vi "功率计测试平台.vi"(11 "Queue Ref In":T1={"UI"=refnum, "Message"=refnum, "Data"=refnum, "Caller"=refnum, "Name"="000 Common", "Data Path"=path "", "Class Path"=path "", "SubPanel"=refnum, "Project Name"="", "MNT"="", "Title"="", "Data Source"=refnum, "Queue List"={}, "VI"=refnum, "UE"=refnum}) -> ()   [LabVIEW 2020]
doc: "000001"
uses:
  Alin/QMH/000 Module Data Type.ctl
  Alin/QMH/Queue Message.ctl
  <vilib>/Utility/NIReport.llb/NI_report.lvclass
  <vilib>/Utility/NIReport.llb/Report Type.ctl
  <vilib>/addons/_office/excel.llb/Excel Easy Table (str).vi
  <vilib>/Utility/NIReport.llb/NI_ReportGenerationCore.lvlib
  <vilib>/Utility/NIReport.llb/Excel/NI_Excel.lvclass
  <vilib>/addons/_office/NI_ReportGenerationToolkit.lvlib
panel:
  out "SN:":string
  out "型号:":string
  in  "Connect":bool
  out "Connected?":bool
  in  "Port":u16 caption="Port:"
  in  "IP:":string
  out "消息":string
  in  "结束":bool
  in  "开始":bool
  in  "时间间隔(s)":dbl=1.0
  out "-W/mW":dbl format="%#.6f W"
  in  "反向通道Offset":dbl min=-60.0 max=60.0 format="%#.2f"
  out "驻波比":dbl format="%#.2f"
  in  "驻波比限值":dbl
  out "W/mW":dbl format="%#.6f W"
  in  "Write":bool
  in  "Read":bool
  in  "正向通道Offset":dbl min=-60.0 max=60.0 format="%#.2f"
  in  "Frequency":dbl=1.0 min=1.0 max=2.0 step=0.1 format="%#.1f GHz"
  out "Channel 1":dbl(knob) scale=0.0..60.0 scale format="%#_2f"
  out "Channel 2":dbl(knob) scale=0.0..60.0 scale format="%#_2f"
  # "Power-CHB"
  # "Power-CHA"
  # "dBm"
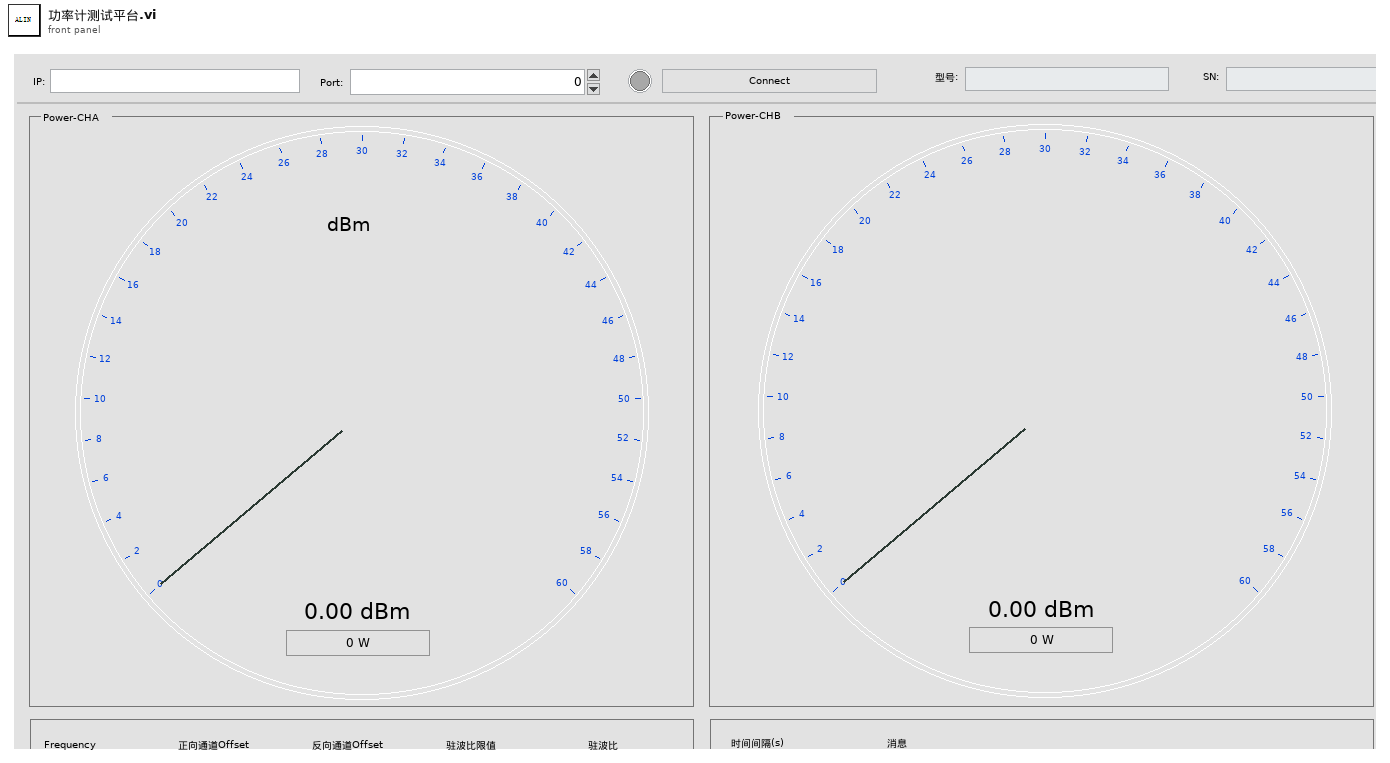
[diagram p1: front panel]
types:
  T1 = typedef "000 Module Data Type.ctl" = cluster{"UI":refnum<queue>, "Message":refnum<queue>, "Data":refnum<queue>, "Caller":refnum<queue>, "Name":string, "Data Path":path, "Class Path":path, "SubPanel":refnum<vi>, "Project Name":string, "MNT":string, "Title":string, "Data Source":refnum<queue>, "Queue List":map{string, refnum<queue>}, "VI":refnum<vi>, "UE":refnum<user-event>}
  T2 = cluster{"Queue":T1, "Delay":cluster{"Count Time(ms)":u32, "Delay Time(ms)":u32, "Next":string}, "connection ID":refnum<k5>, "Save path":path, "report":refnum<class "NI_report.lvclass">, "Count":u32}
  T3 = typedef "NI_ReportGenerationCore.lvlib/Report Type.ctl" = enum16{"HTML", "Word", "Excel"}
  T4 = enum16{"maximized", "minimized", "normal", "no change"}
  T5 = typedef "eventvkey.ctl" = enum16{"ASCII", "Enter", "Return", "Shift", "Ctrl", "Alt", "Cmd", "Opt", "Caps", "NumLock", "Clear", "Break", "Up", "Down", "Left", "Right", "Insert", "Delete", "Home", "End", "PageUp", "PageDown", "Escape", "Help", "Pause", "ScrollLock", "F1", "F2", "F3", "F4", "F5", "F6", "F7", "F8", "F9", "F10", "F11", "F12", "F13", "F14", "F15", "F16", "F17", "F18", "F19", "F20", "F21", "F22", "F23", "F24", "Play", "VolumeUp", "VolumeDown", "Mute", "Two Byte Char"}
  T6 = cluster{"Shift":bool, "Ctrl":bool, "Alt":bool, "Cmd":bool, "Opt":bool}
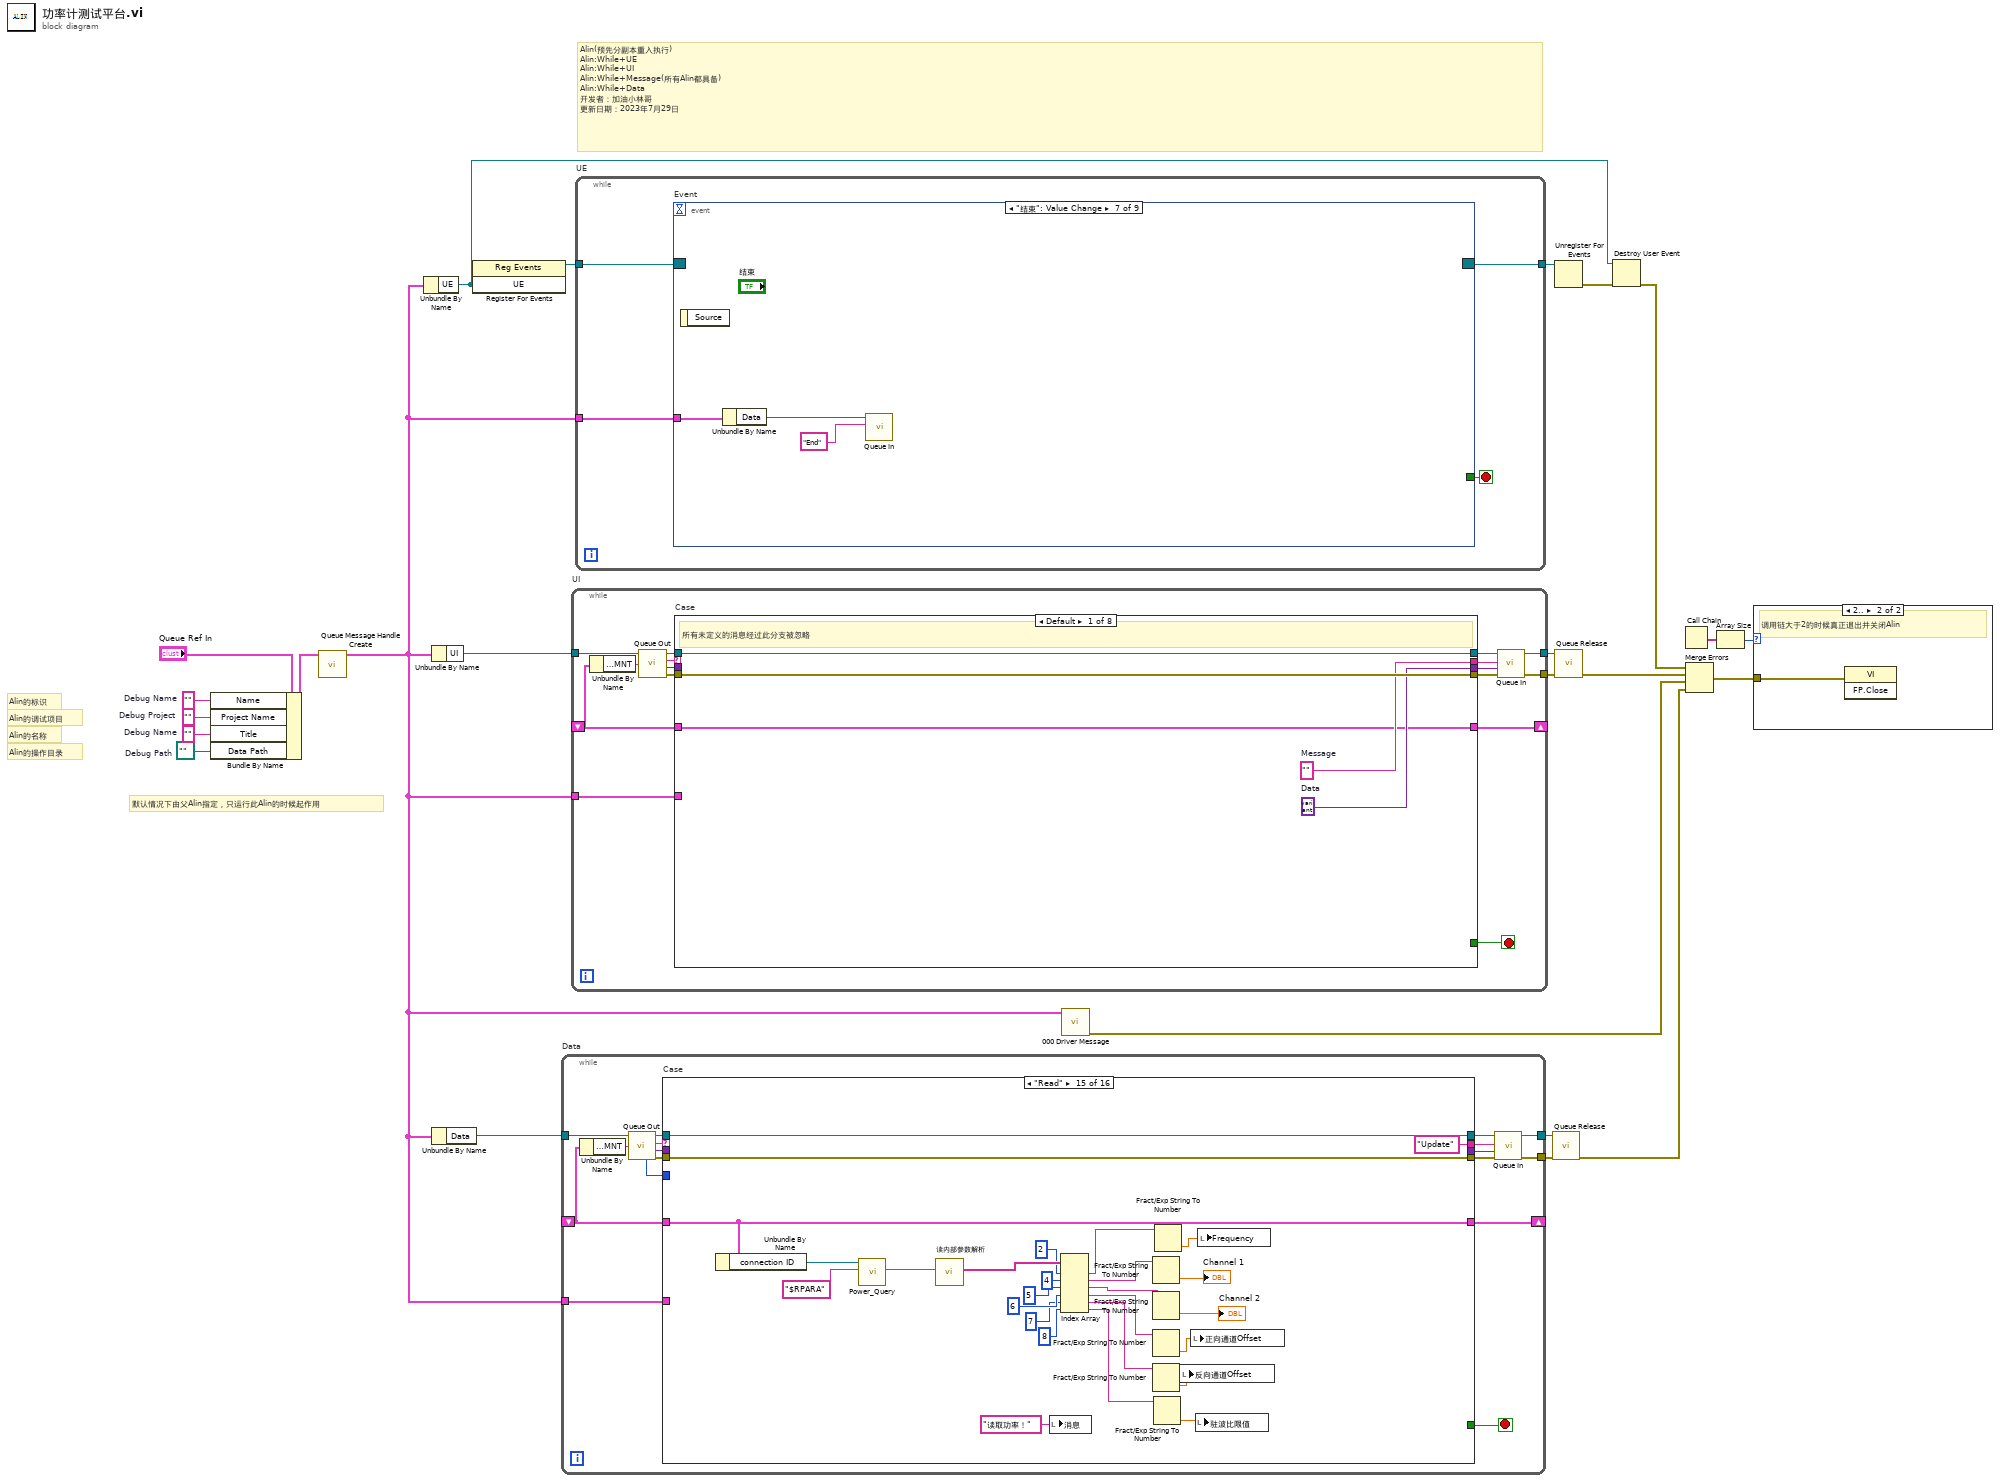
[diagram p0: block diagram]
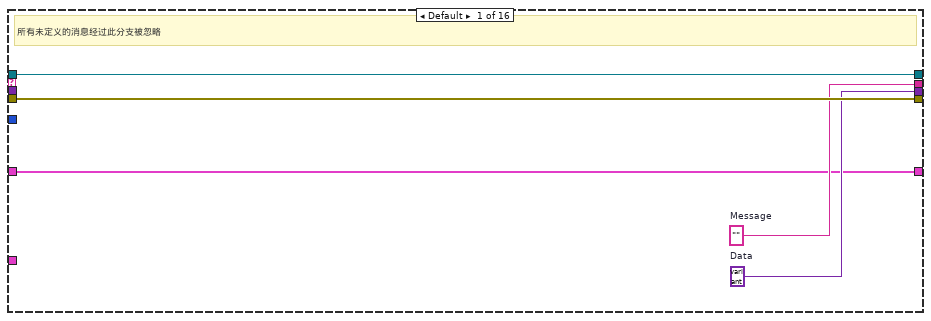
[diagram p2: hidden frame]
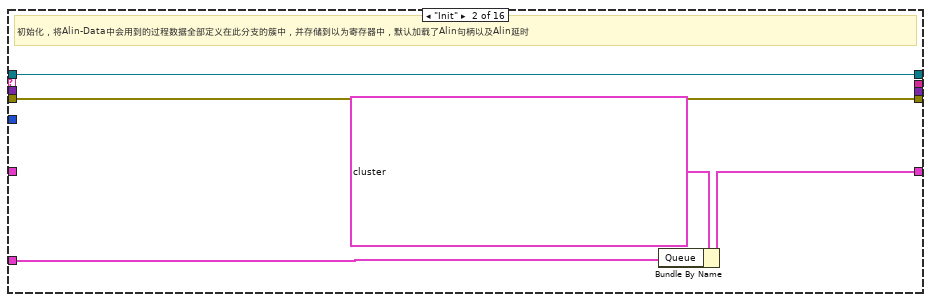
[diagram p3: hidden frame]
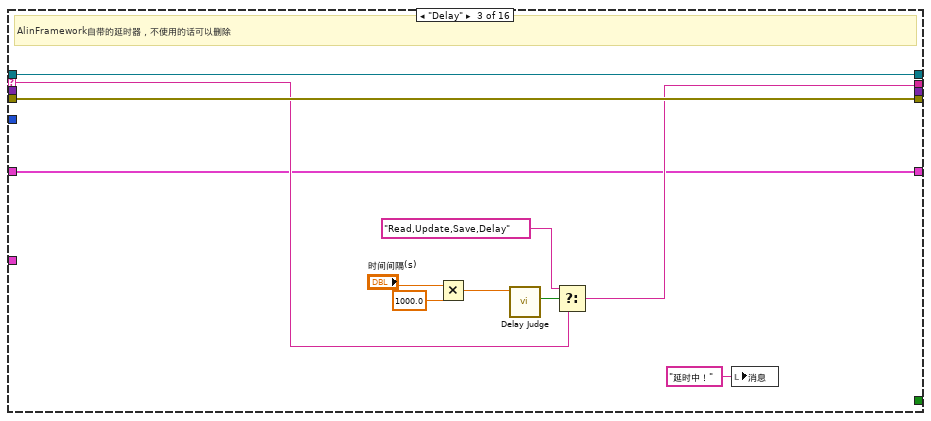
[diagram p4: hidden frame]
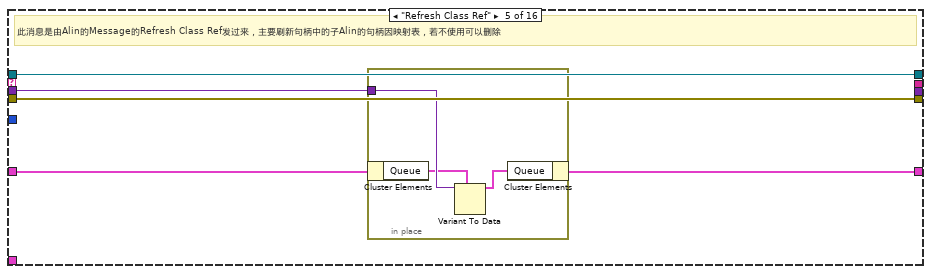
[diagram p6: hidden frame]
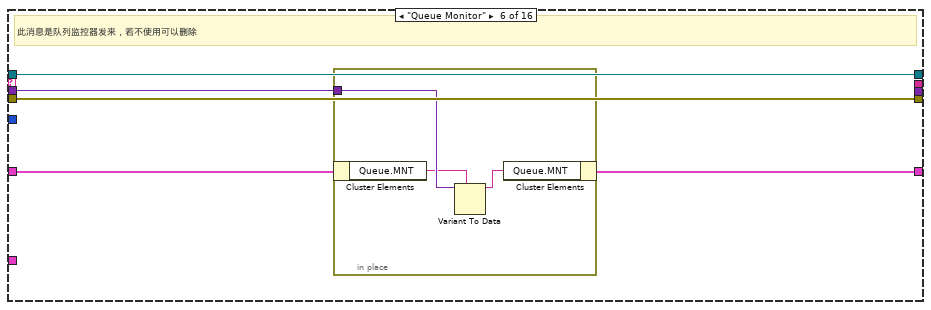
[diagram p7: hidden frame]
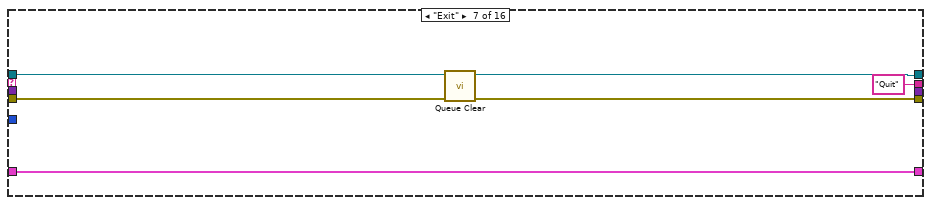
[diagram p8: hidden frame]
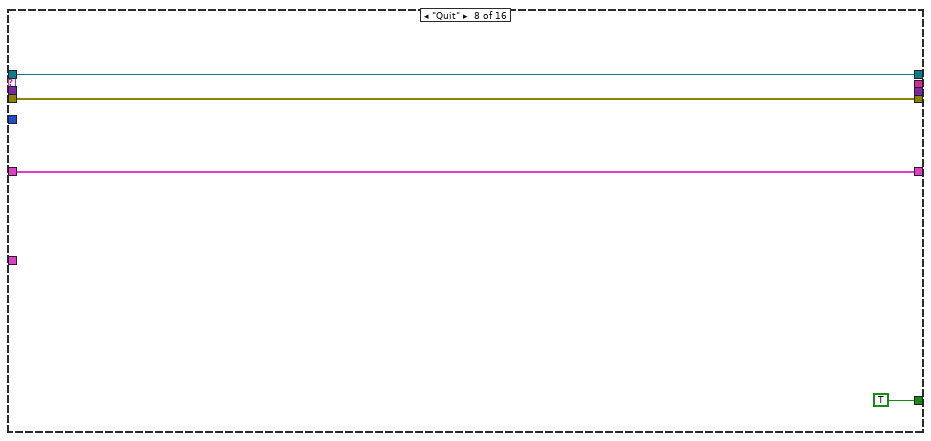
[diagram p9: hidden frame]
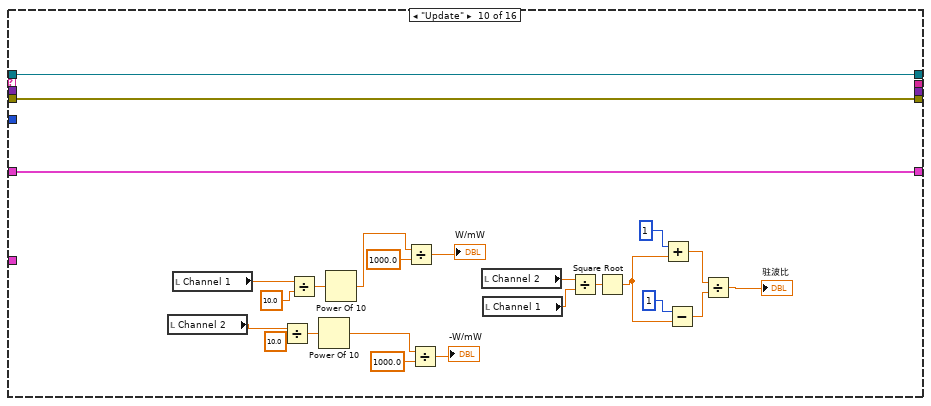
[diagram p11: hidden frame]
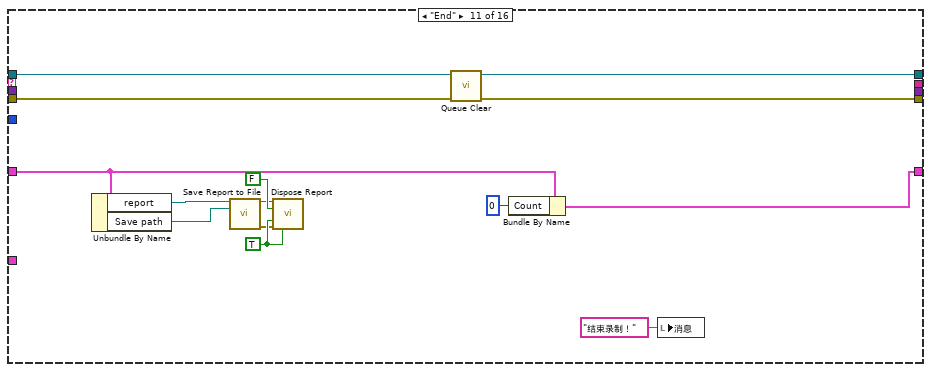
[diagram p12: hidden frame]
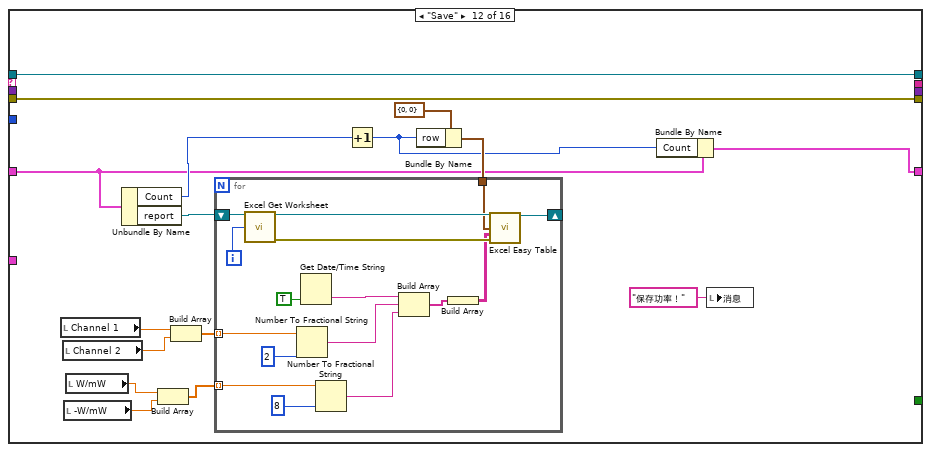
[diagram p13: hidden frame]
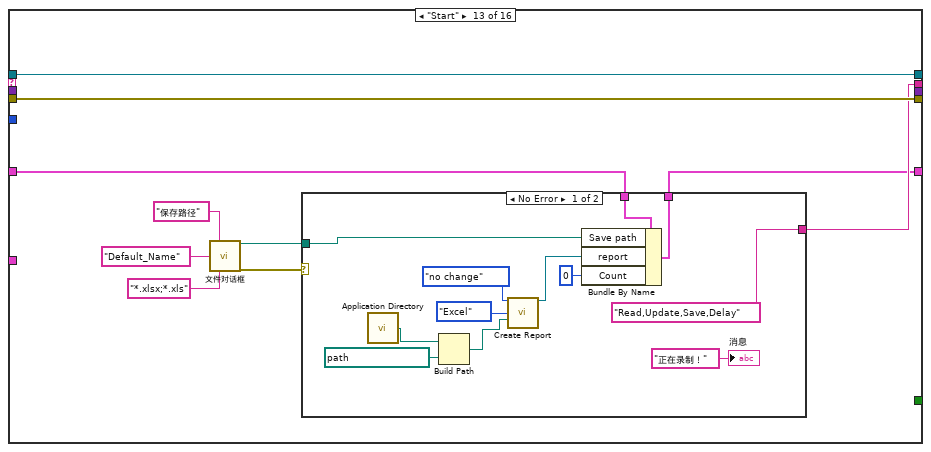
[diagram p14: hidden frame]
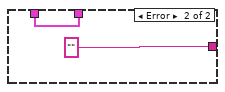
[diagram p15: hidden frame]
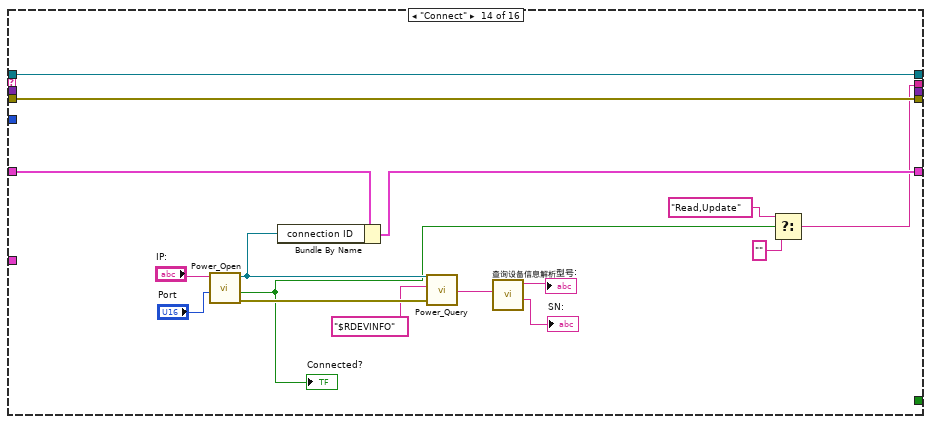
[diagram p16: hidden frame]
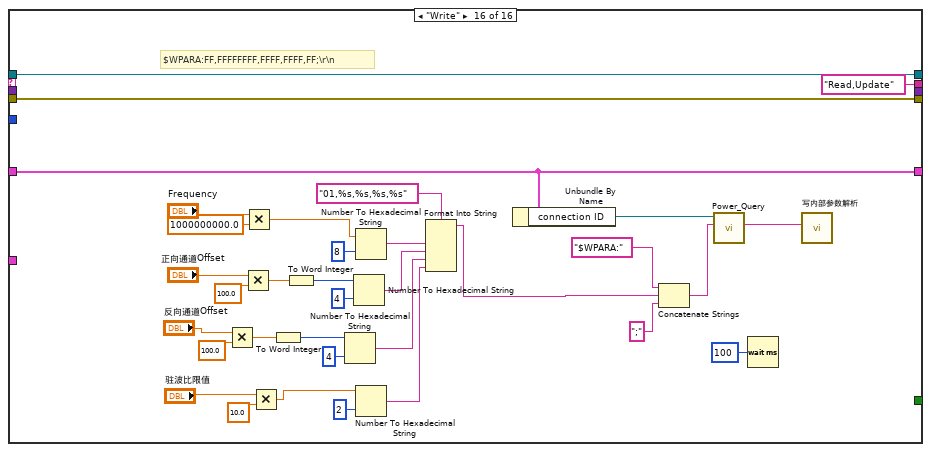
[diagram p17: hidden frame]
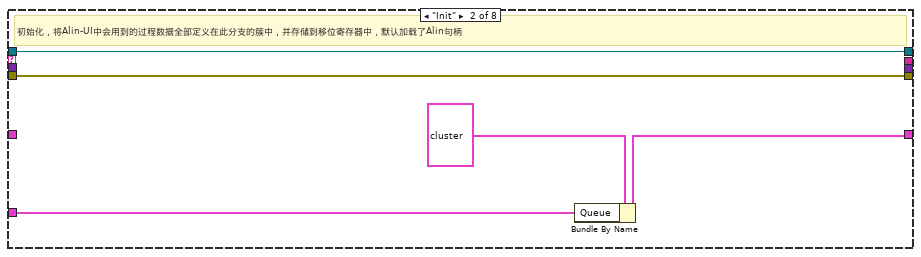
[diagram p19: hidden frame]
diagram:
  w1 = ""  # Debug Name
  w2 = ""  # Debug Project
  w3 = path ""  # Debug Path
  w4 = ""  # Debug Name
  # "Alin(预先分副本重入执行)\nAlin:While+UE\nAlin:While+UI\nAlin:While+Message(所有Alin都具备)\nAlin:While+Data\n开发者：加油小林哥\n更新日期：2023年7月29日"
  # "默认情况下由父Alin指定，只运行此Alin的时候起作用"
  # "Alin的标识"
  # "Alin的调试项目"
  # "Alin的名称"
  # "Alin的操作目录"
  n1 = Bundle By Name ("按名称捆绑")(cluster="Queue Ref In", "Name"=w1, "Project Name"=w2, "Title"=w4, "Data Path"=w3) -> (w5:T1)
  n2 = call "Queue Message Handle Create.vi"("Queue Ref In"=w5) -> ("Queue Ref Out"=w6:T1)  [unwired: 8 in, 2 out]
  n3 = Unbundle By Name ("按名称解除捆绑")(w6) -> ("UE"=w8:refnum<user-event>)
  n4 = Unbundle By Name ("按名称解除捆绑")(w6) -> ("UI"=w19:refnum<queue>)
  n5 = Unbundle By Name ("按名称解除捆绑")(w6) -> ("Data"=w11:refnum<queue>)
  n6 = register-events ("注册事件")(w8) -> (reference out=w24:refnum<event-registration>)  [unwired: 2 in, 1 out]
  n7 = while "Data" {
    tunnel: w11 -> [w37]
    tunnel: [w34] -> w13
    tunnel: [w33] -> w12
    shift-right: [w29] -> _
    shift-left: _ -> [w26]
    tunnel: w6 -> [w25]
    stop <- w41 stop-if-true
    n8 = Unbundle By Name ("按名称解除捆绑")(w26) -> ("Queue.MNT"=w27:string)
    n9 = call "Queue Out.vi"("Monitor"=w27, "Queue In"=w37) -> ("error out"=w40:errorcluster, "Data"=w38:variant, "Message"=w39:string, "Queue Out"=w36:refnum<queue>, "Queue NUmber"=w28:i32)  [unwired: 5 in]
    n10 = case "Case" shown="\"Read\"" w39 {
      selector: w39 -> [_ _ w58 _ _ _ _ _ _ _ _ _ _ _ _ _]
      tunnel: w36 -> [w46 w51 w62 w65 w70 w78 w86 w90 w94 w118 w132 w148 w174 w204 w231 w265]
      tunnel: w40 -> [w45 w50 w61 w64 w69 w77 w84 w91 w93 w117 w131 w147 w173 w203 w230 w264]
      tunnel: [w46 w51 w62 w65 w70 w78 w85 w90 w94 w118 w129 w148 w174 w204 w231 w265] -> w35
      tunnel: [w45 w50 w61 w64 w69 w77 w83 w91 w93 w117 w130 w147 w173 w203 w230 w264] -> w32
      tunnel: [w44 _ w59 _ _ _ "Quit" _ _ _ _ _ w167 w189 "Update" ("CMD") "Read,Update" ("CMD")] -> w31
      tunnel: [_ _ _ _ _ _ _ TRUE _ _ _ _ _ _ _ _] -> w41
      tunnel: [w43 _ _ _ _ _ _ _ _ _ _ _ _ _ _ _] -> w30
      tunnel: w38 -> [_ _ _ _ w66 w74 _ _ _ _ _ _ _ _ _ _]
      tunnel: [w42 w48 w57 w63 w67 w75 w82 w88 w92 w116 w120 w135 w165 w199 w229 w263] -> w29
      tunnel: w26 -> [w42 _ w57 w63 w68 w76 w82 w88 w92 w116 w122 w136 w166 w200 w229 w263]
      tunnel: w28 -> [_ _ _ _ _ _ _ _ _ _ _ _ _ _ _ _]
      tunnel: w25 -> [_ w47 _ _ _ _ _ _ _ _ _ _ _ _ _ _]
      frame Default {
        w43 = variant  # Data
        w44 = ""  # Message
        # "所有未定义的消息经过此分支被忽略"
      }
      frame "Init" {
        # "初始化，将Alin-Data中会用到的过程数据全部定义在此分支的簇中，并存储到以为寄存器中，默认加载了Alin句柄以及Alin延时"
        n11 = Bundle By Name(cluster=T2 {"Queue"={"UI"=refnum, "Message"=refnum, "Data"=refnum, "Caller"=refnum, "Name"="000 Common", "Data Path"=path "", "Class Path"=path "", "SubPanel"=refnum, "Project Name"="", "MNT"="", "Title"="", "Data Source"=refnum, "Queue List"={}, "VI"=refnum, "UE"=refnum}, "Delay"={"Count Time(ms)"=250, "Delay Time(ms)"=250, "Next"="Receive Data,Delay"}, "connection ID"=refnum, "Save path"=path "", "report"=refnum, "Count"=250}, "Queue"=w47) -> (w48:T2)
      }
      frame "Delay" {
        # "AlinFramework自带的延时器，不使用的话可以删除"
        n12 = Multiply(x="时间间隔(s)", y=1000.0) -> (x*y=w54:dbl)
        n13 = call "Delay Judge.vi"("Count Time(ms)"=w54) -> ("Time Out?"=w60:bool)  [unwired: 6 in, 4 out]
        n14 = Select(t="Read,Update,Save,Delay", s=w60, f=w58) -> (s? t:f=w59:string)
        n15 = local write "消息"("延时中！" ("消息")) -> ()
      }
      frame "====System====" {
      }
      frame "Refresh Class Ref" {
        # "此消息是由Alin的Message的Refresh Class Ref发过来，主要刷新句柄中的子Alin的句柄因映射表，若不使用可以删除"
        n16 = in-place {
          in-place-border: w66 -> [w73]
          n17 = in-place-cluster #1(w68) -> ("Queue"=w72:T1)
          n18 = Variant To Data(type=w72, Variant=w73) -> (data=w71:T1)  [unwired: 1 in, 1 out]
          n19 = in-place-cluster #1("Queue"=w71) -> (w67:T2)
        }
      }
      frame "Queue Monitor" {
        # "此消息是队列监控器发来，若不使用可以删除"
        n20 = in-place {
          in-place-border: w74 -> [w81]
          n21 = in-place-cluster #2(w76) -> ("Queue.MNT"=w80:string)
          n22 = Variant To Data(type=w80, Variant=w81) -> (data=w79:string)  [unwired: 1 in, 1 out]
          n23 = in-place-cluster #2("Queue.MNT"=w79) -> (w75:T2)
        }
      }
      frame "Exit" {
        n24 = call "Queue Clear.vi"("error in (no error)"=w84, "Queue In"=w86) -> ("error out"=w83:errorcluster, "Queue Out"=w85:refnum<queue>)  [unwired: 8 in]
      }
      frame "Quit" {
      }
      frame "====User====" {
      }
      frame "Update" {
        n25 = local read "Channel 2"() -> (w112:dbl)
        n26 = local read "Channel 1"() -> (w114:dbl)
        n27 = Divide(x=w112, y=10.0) -> (x/y=w113:dbl)
        n28 = Divide(x=w114, y=10.0) -> (x/y=w115:dbl)
        n29 = Power Of 10(x=w113) -> (10^x=w106:dbl)
        n30 = Power Of 10(x=w115) -> (10^x=w109:dbl)
        n31 = Divide(x=w109, y=1000.0) -> (x/y=→"W/mW":dbl)
        n32 = Divide(x=w106, y=1000.0) -> (x/y=→"-W/mW":dbl)
        n33 = local read "Channel 2"() -> (w98:dbl)
        n34 = local read "Channel 1"() -> (w97:dbl)
        n35 = Divide(x=w98, y=w97) -> (x/y=w103:dbl)
        n36 = Square Root(x=w103) -> (sqrt(x)=w96:dbl)
        n37 = Add(x=1, y=w96) -> (x+y=w101:dbl)
        n38 = Subtract(x=1, y=w96) -> (x-y=w102:dbl)
        n39 = Divide(x=w101, y=w102) -> (x/y=→"驻波比":dbl)
      }
      frame "End" {
        w128 = TRUE ("save changes? (F)")
        n40 = Unbundle By Name(w122) -> ("report"=w124:refnum<class "NI_report.lvclass">, "Save path"=w123:path)
        n41 = call-dynamic "Save Report to File.vi"("report in"=w124, "report file path"=w123) -> ("report out"=w125:refnum<class "NI_report.lvclass">, "error out"=w126:errorcluster)  [unwired: 12 in]
        n42 = call-dynamic "Dispose Report.vi"("report in"=w125, "wait until printing completed? (T)"=FALSE, "save changes? (F)"=w128, "error in (no error)"=w126, "close report? (T)"=w128) -> ()  [unwired: 10 in, 1 out]
        n43 = call "Queue Clear.vi"("error in (no error)"=w131, "Queue In"=w132) -> ("error out"=w130:errorcluster, "Queue Out"=w129:refnum<queue>)  [unwired: 8 in]
        n44 = Bundle By Name(cluster=w122, "Count"=u32 0) -> (w120:T2)
        n45 = local write "消息"("结束录制！" ("消息")) -> ()
      }
      frame "Save" {
        n46 = local read "Channel 1"() -> (w145:dbl)
        n47 = local read "Channel 2"() -> (w144:dbl)
        n48 = local read "-W/mW"() -> (w142:dbl)
        n49 = local read "W/mW"() -> (w143:dbl)
        n50 = Unbundle By Name(w136) -> ("Count"=w139:u32, "report"=w146:refnum<class "NI_report.lvclass">)
        n51 = Build Array(w143, w142) -> (w140:dbl[])
        n52 = Build Array(w145, w144) -> (w141:dbl[])
        n53 = Increment(x=w139) -> (x+1=w134:u32)
        n54 = Bundle By Name(cluster=cluster{"row":i32, "column":i32} {"row"=0, "column"=0} ("start (0, 0)"), "row"=w134) -> (w137:cluster{"row":i32, "column":i32})
        n55 = for {
          tunnel: w141 -> [w152] mode=indexing
          tunnel: w140 -> [w151] mode=indexing
          shift-right: [w150] -> _
          shift-left: w146 -> [w164]
          tunnel: w137 -> [w149]
          i -> [w153]
          n56 = call <vilib>:"Excel Get Worksheet.vi"("report in"=w164, "worksheet index (0)"=w153) -> ("report out"=w162:refnum<class "NI_report.lvclass">, "error out"=w163:errorcluster)  [unwired: 12 in]
          n57 = Number To Fractional String(number=w152, precision (6)=i16 2) -> (F-format string=w158:string)  [unwired: 2 in]
          n58 = Get Date/Time String(want seconds? (F)=TRUE) -> (time string=w160:string)  [unwired: 2 in, 1 out]
          n59 = Number To Fractional String(number=w151, precision (6)=i16 8) -> (F-format string=w156:string)  [unwired: 2 in]
          n60 = Build Array(w160, w158, w156) -> (w155:string[])
          n61 = Build Array(w155) -> (w154:string[][])
          n62 = call-poly <vilib>:"Excel Easy Table.vi"("report in"=w162, "start (0, 0)"=w149, "text data"=w154, "error in (no error)"=w163) -> ("report out"=w150:refnum<class "NI_report.lvclass">)  [unwired: 7 in, 4 out]
        }
        n63 = Bundle By Name(cluster=w136, "Count"=w134) -> (w135:T2)
        n64 = local write "消息"("保存功率！" ("消息")) -> ()
      }
      frame "Start" {
        n65 = call "文件对话框"("prompt"="保存路径" ("default name"), "default name"="Default_Name", "pattern (all files)"="*.xlsx;*.xls") -> ("selected path"=w172:path, "error out"=w171:errorcluster)  [unwired: 9 in, 2 out]
        n66 = case shown="No Error" w171 {
          tunnel: w172 -> [w183 _]
          tunnel: ["Read,Update,Save,Delay" ""] -> w167
          tunnel: w166 -> [w184 w187]
          tunnel: [w182 w187] -> w165
          frame No Error {
            n67 = call <vilib>:"Application Directory.vi"() -> ("Application Directory"=w181:path)
            n68 = Build Path(base path=w181, name or relative path=path "Config/模版.xlsx") -> (appended path=w179:path)
            n69 = call <vilib>:"Create Report.vi"("window state (normal)"=T4."no change", "report type"=Report_Type."Excel", "template (empty)"=w179) -> ("report out"=w178:refnum<class "NI_report.lvclass">)  [unwired: 11 in, 1 out]
            n70 = Bundle By Name(cluster=w184, "Save path"=w183, "report"=w178, "Count"=u32 0) -> (w182:T2)
            "消息" <- "正在录制！" ("消息")
          }
          frame Error {
          }
        }
      }
      frame "Connect" {
        n71 = call "Power_Open.vi"("Port"="Port", "IP:"="IP:") -> ("error out"=w197:errorcluster, "Connected?"=w192:bool, "connection ID"=w198:refnum<k5>)  [unwired: 7 in]
        "Connected?" <- w192
        n72 = Bundle By Name(cluster=w200, "connection ID"=w198) -> (w199:T2)
        n73 = call "Power_Query.vi"("error in (no error)"=w197, "CMD"="$RDEVINFO", "connection ID"=w198) -> ("Read Buffer"=w195:string)  [unwired: 6 in, 2 out]
        n74 = call "查询设备信息解析.vi"("响应"=w195) -> ("SN"=→"SN:":string, "型号"=→"型号:":string)  [unwired: 9 in]
        n75 = Select(t="Read,Update" ("CMD"), s=w192, f="" ("CMD")) -> (s? t:f=w189:string)
      }
      frame "Read" {
        n76 = Unbundle By Name(w229) -> ("connection ID"=w228:refnum<k5>)
        n77 = call "Power_Query.vi"("CMD"="$RPARA", "connection ID"=w228) -> ("Read Buffer"=w226:string)  [unwired: 7 in, 2 out]
        n78 = call "读内部参数解析.vi"("响应"=w226) -> ("读内部参数"=w225:string[])  [unwired: 10 in]
        n79 = local write "消息"("读取功率！" ("消息")) -> ()
        n80 = Index Array(array=w225, index #1=2 ("index"), index #2=4 ("index"), index #3=5 ("index"), index #4=6 ("index"), index #5=7 ("index"), index #6=8 ("index")) -> (element #1=w209:string, element #2=w222:string, element #3=w220:string, element #4=w217:string, element #5=w216:string, element #6=w212:string)
        n81 = Fract/Exp String To Number(string=w222) -> (number=→"Channel 1":dbl)  [unwired: 3 in, 1 out]
        n82 = Fract/Exp String To Number(string=w220) -> (number=→"Channel 2":dbl)  [unwired: 3 in, 1 out]
        n83 = Fract/Exp String To Number(string=w217) -> (number=w215:dbl)  [unwired: 3 in, 1 out]
        n84 = Fract/Exp String To Number(string=w216) -> (number=w214:dbl)  [unwired: 3 in, 1 out]
        n85 = Fract/Exp String To Number(string=w212) -> (number=w211:dbl)  [unwired: 3 in, 1 out]
        n86 = Fract/Exp String To Number(string=w209) -> (number=w208:dbl)  [unwired: 3 in, 1 out]
        n87 = local write "反向通道Offset"(w214) -> ()
        n88 = local write "正向通道Offset"(w215) -> ()
        n89 = local write "驻波比限值"(w211) -> ()
        n90 = local write "Frequency"(w208) -> ()
      }
      frame "Write" {
        # "$WPARA:FF,FFFFFFFF,FFFF,FFFF,FF;\\r\\n"
        n91 = Multiply(x="反向通道Offset", y=100.0) -> (x*y=w247:dbl)
        n92 = Multiply(x="正向通道Offset", y=100.0) -> (x*y=w255:dbl)
        n93 = Multiply(x="Frequency", y=1000000000.0) -> (x*y=w234:dbl)
        n94 = Multiply(x="驻波比限值", y=10.0) -> (x*y=w239:dbl)
        n95 = To Word Integer(number=w247) -> (16bit integer=w243:i16)
        n96 = To Word Integer(number=w255) -> (16bit integer=w244:i16)
        n97 = Number To Hexadecimal String(1:i16 4 ("width (-)"), 2:w243) -> (0:w245:string)
        n98 = Number To Hexadecimal String(1:i16 4 ("width (-)"), 2:w244) -> (0:w254:string)
        n99 = Number To Hexadecimal String(1:i16 8 ("宽度(-)"), 2:w234) -> (0:w257:string)
        n100 = Number To Hexadecimal String(1:i16 2 ("width (-)"), 2:w239) -> (0:w238:string)
        n101 = Format Into String(format string="01,%s,%s,%s,%s" ("string"), w257, w254, w245, w238) -> (resulting string=w237:string)  [unwired: 2 in, 1 out]
        n102 = Unbundle By Name(w263) -> ("connection ID"=w262:refnum<k5>)
        n103 = Concatenate Strings("$WPARA:" ("CMD"), w237, ";" ("string")) -> (w259:string)
        n104 = call "Power_Query.vi"("CMD"=w259, "connection ID"=w262) -> ("Read Buffer"=w258:string)  [unwired: 7 in, 2 out]
        n105 = Wait (ms)(milliseconds to wait=u32 100) -> ()  [unwired: 1 out]
        n106 = call "写内部参数解析.vi"("响应"=w258) -> ()  [unwired: 10 in, 1 out]
      }
    }
    n107 = call "Queue In.vi"("error in (no error)"=w32, "Data"=w30, "Message"=w31, "Queue In"=w35) -> ("error out"=w33:errorcluster, "Queue Out"=w34:refnum<queue>)  [unwired: 6 in]
  }
  n108 = while "UI" {
    tunnel: w19 -> [w277]
    tunnel: [w274] -> w21
    tunnel: [w273] -> w20
    shift-right: [w269] -> _
    shift-left: _ -> [w268]
    tunnel: w6 -> [w266]
    stop <- w281 stop-if-true
    n109 = Unbundle By Name ("按名称解除捆绑")(w268) -> ("Queue.MNT"=w267:string)
    n110 = call "Queue Out.vi"("Monitor"=w267, "Queue In"=w277) -> ("error out"=w280:errorcluster, "Data"=w278:variant, "Message"=w279:string, "Queue Out"=w276:refnum<queue>)  [unwired: 5 in, 1 out]
    n111 = case "Case" shown="Default" w279 {
      tunnel: w276 -> [w286 w291 w294 w299 w307 w315 w319 w323]
      tunnel: w280 -> [w285 w290 w293 w298 w306 w313 w320 w322]
      tunnel: [w286 w291 w294 w299 w307 w314 w319 w323] -> w275
      tunnel: [w285 w290 w293 w298 w306 w312 w320 w322] -> w272
      tunnel: [w284 _ _ _ _ "Quit" _ _] -> w271
      tunnel: [_ _ _ _ _ _ TRUE _] -> w281
      tunnel: [w283 _ _ _ _ _ _ _] -> w270
      tunnel: w278 -> [_ _ _ w295 w303 _ _ _]
      tunnel: [w282 w288 w292 w296 w304 w311 w317 w321] -> w269
      tunnel: w268 -> [w282 _ w292 w297 w305 w311 w317 w321]
      tunnel: w266 -> [_ w287 _ _ _ _ _ _]
      frame Default {
        w283 = variant  # Data
        w284 = ""  # Message
        # "所有未定义的消息经过此分支被忽略"
      }
      frame "Init" {
        # "初始化，将Alin-UI中会用到的过程数据全部定义在此分支的簇中，并存储到移位寄存器中，默认加载了Alin句柄"
        n112 = Bundle By Name(cluster=cluster{"Queue":T1} {"Queue"={"UI"=refnum, "Message"=refnum, "Data"=refnum, "Caller"=refnum, "Name"="000 Common", "Data Path"=path "", "Class Path"=path "", "SubPanel"=refnum, "Project Name"="", "MNT"="", "Title"="", "Data Source"=refnum, "Queue List"={}, "VI"=refnum, "UE"=refnum}}, "Queue"=w287) -> (w288:cluster{"Queue":T1})
      }
      frame "====System====" {
      }
      frame "Refresh Class Ref" {
        # "此消息是由Alin的Message的Refresh Class Ref发过来，主要刷新句柄中的子Alin的句柄因映射表，若不使用可以删除"
        n113 = in-place {
          in-place-border: w295 -> [w302]
          n114 = in-place-cluster #3(w297) -> ("Queue"=w301:T1)
          n115 = Variant To Data(type=w301, Variant=w302) -> (data=w300:T1)  [unwired: 1 in, 1 out]
          n116 = in-place-cluster #3("Queue"=w300) -> (w296:cluster{"Queue":T1})
        }
      }
      frame "Queue Monitor" {
        # "此消息是队列监控器发来，若不使用可以删除"
        n117 = in-place {
          in-place-border: w303 -> [w310]
          n118 = in-place-cluster #4(w305) -> ("Queue.MNT"=w309:string)
          n119 = Variant To Data(type=w309, Variant=w310) -> (data=w308:string)  [unwired: 1 in, 1 out]
          n120 = in-place-cluster #4("Queue.MNT"=w308) -> (w304:cluster{"Queue":T1})
        }
      }
      frame "Exit" {
        n121 = call "Queue Clear.vi"("error in (no error)"=w313, "Queue In"=w315) -> ("error out"=w312:errorcluster, "Queue Out"=w314:refnum<queue>)  [unwired: 8 in]
      }
      frame "Quit" {
      }
      frame "====User====" {
      }
    }
    n122 = call "Queue In.vi"("error in (no error)"=w272, "Data"=w270, "Message"=w271, "Queue In"=w275) -> ("error out"=w273:errorcluster, "Queue Out"=w274:refnum<queue>)  [unwired: 6 in]
  }
  n123 = while "UE" {
    tunnel: w24 -> [w327]
    tunnel: [w325] -> w23
    tunnel: w6 -> [w324]
    stop <- w326 stop-if-true
    n124 = event "Event" shown="[6] \"结束\": Value Change" {
      selector: w327 -> [_ _ _ _ _ _ _ _ _]
      dyn-events: [_ _ _ _ _ _ _ _ _] -> w325
      timeout: _ -> [_ _ _ _ _ _ _ _ _]
      tunnel: [_ _ _ _ _ _ _ w348 _] -> w326
      tunnel: w324 -> [_ w328 w335 w338 w341 w344 w347 _ w353]
      event Timeout {
        n125 = event-data() -> ()  [unwired: 1 in, 1 out]
      }
      event Key Down {
        # "所有界面上按键按下事件的处理"
        n126 = event-data() -> ("Char"=w331:i16, "VKey"=w332:T5, "Mods"=w330:cluster{"Num Pad":bool, "Menu Key":bool}, "PlatMods"=w329:T6)  [unwired: 1 in]
        n127 = call "Queue Key Down.vi"("Queue Ref Out"=w328, "C"=w331, "Platform Key"=w329, "Group Key"=w330, "V Key"=w332) -> ()  [unwired: 6 in, 1 out]
      }
      event "Connect": Value Change {
        n128 = event-data() -> ()  [unwired: 1 in, 1 out]
        n129 = Unbundle By Name ("按名称解除捆绑")(w335) -> ("Data"=w334:refnum<queue>)
        n130 = call "Queue In.vi"("Message"="Connect", "Queue In"=w334) -> ()  [unwired: 8 in, 2 out]
      }
      event "Read": Value Change {
        n131 = event-data() -> ()  [unwired: 1 in, 1 out]
        n132 = Unbundle By Name ("按名称解除捆绑")(w338) -> ("Data"=w337:refnum<queue>)
        n133 = call "Queue In.vi"("Message"="Read", "Queue In"=w337) -> ()  [unwired: 8 in, 2 out]
      }
      event "Write": Value Change {
        n134 = event-data() -> ()  [unwired: 1 in, 1 out]
        n135 = Unbundle By Name ("按名称解除捆绑")(w341) -> ("Data"=w340:refnum<queue>)
        n136 = call "Queue In.vi"("Message"="Write", "Queue In"=w340) -> ()  [unwired: 8 in, 2 out]
      }
      event "开始": Value Change {
        n137 = event-data() -> ()  [unwired: 1 in, 1 out]
        n138 = Unbundle By Name ("按名称解除捆绑")(w344) -> ("Data"=w343:refnum<queue>)
        n139 = call "Queue In.vi"("Message"="Start", "Queue In"=w343) -> ()  [unwired: 8 in, 2 out]
      }
      event "结束": Value Change {
        n140 = event-data() -> ()  [unwired: 1 in, 1 out]
        n141 = Unbundle By Name ("按名称解除捆绑")(w347) -> ("Data"=w346:refnum<queue>)
        n142 = call "Queue In.vi"("Message"="End", "Queue In"=w346) -> ()  [unwired: 8 in, 2 out]
      }
      event User Event {
        # "此分支有Alin的Message线程发送过来用来退出用户事件所在的线程"
        n143 = event-data() -> ("Message"=w350:string)  [unwired: 1 in]
        n144 = Equal?(x=w350, y="Exit") -> (x = y?=w348:bool)
      }
      event Panel Close? {
        # "用户点击前面板关闭的按键"
        n145 = event-data() -> ()  [unwired: 1 in, 1 out]
        n146 = Call Chain() -> (call chain=w355:string[])
        n147 = Array Size(array=w355) -> (size(s)=w354:i32)
        n148 = case shown="2, Default" w354 {
          tunnel: w353 -> [w359 w362]
          tunnel: [w358 w361] -> w352
          tunnel: ["Panel Hidden" ("Message") "Exit Prepare" ("Message")] -> w351
          frame 2, Default {
            # "当调用链大于2的时候，只隐藏前面板"
            n149 = Unbundle By Name(w359) -> ("Message"=w358:refnum<queue>)
          }
          frame 1 {
            # "只打开此Alin的时候使用默认退出"
            n150 = Unbundle By Name(w362) -> ("Message"=w361:refnum<queue>)
          }
        }
        n151 = call "Queue In.vi"("Message"=w351, "Queue In"=w352) -> ()  [unwired: 8 in, 2 out]
        n152 = event-data("Discard?"=TRUE ("放弃？")) -> ()  [unwired: 1 in, 1 out]
      }
    }
  }
  n153 = call "000 Driver Message.vi"("Queue In"=w6) -> ("error out"=w9:errorcluster)  [unwired: 8 in, 2 out]
  n154 = call "Queue Release.vi"("error in (no error)"=w12, "Queue In"=w13) -> ("error out"=w10:errorcluster)  [unwired: 9 in]
  n155 = Unregister For Events ("取消注册事件")(event registration refnum=w23) -> (error out=w22:errorcluster)  [unwired: 1 in]
  n156 = call "Queue Release.vi"("error in (no error)"=w20, "Queue In"=w21) -> ("error out"=w17:errorcluster)  [unwired: 9 in]
  n157 = Destroy User Event ("销毁用户事件")(user event=w8, error in=w22) -> (error out=w18:errorcluster)
  n158 = Call Chain ("调用链")() -> (call chain=w15:string[])
  n159 = Merge Errors ("合并错误")(w18, w17, w9, w10) -> (w16:errorcluster)
  n160 = Array Size ("数组大小")(array=w15) -> (size(s)=w14:i32)
  n161 = case "条件结构" shown="2.." w14 {
    tunnel: w16 -> [_ w363]
    frame 0, Default {
      # "只运行此Alin的时候不关闭前面面(调试使用)"
    }
    frame 2.. {
      # "调用链大于2的时候真正退出并关闭Alin"
      n162 = invoke class="VI" method="FP.Close"(error in=w363) -> ()  [unwired: 2 in, 3 out]
    }
  }
